vi "Build DB Connection String.vi"(8 "Error In":errorcluster) -> (0 "Error Out":errorcluster, 2 "Database Connection String":string)   [LabVIEW 2013, in "VIChallenge.lvlib"]
uses:
  VIChallenge.lvlib
  <vilib>/Utility/config.llb/Read Key (String).vi
  <vilib>/Utility/config.llb/NI_LVConfig.lvlib
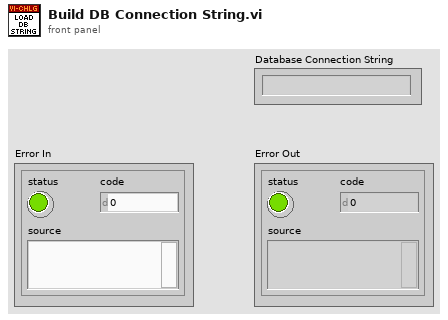
[diagram p1: front panel]
types:
  T1 = typedef "NI_LVConfig.lvlib/Config Data RefNum.ctl" = refnum<k1>
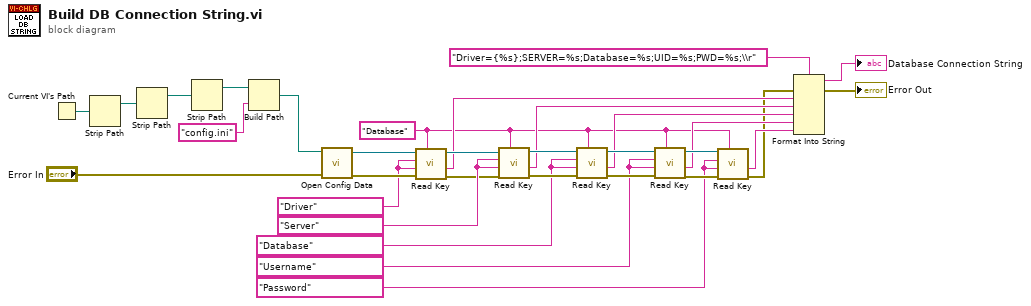
[diagram p0: block diagram]
diagram:
  w8 = "Password"
  w26 = "Username"
  w27 = "Database"
  w28 = "Server"
  w29 = "Driver"
  w3 = "Database" ("section")
  n1 = Current VI's Path() -> (path=w2:path)
  n2 = Strip Path(path=w2) -> (stripped path=w1:path)  [unwired: 1 out]
  n3 = Strip Path(path=w1) -> (stripped path=w20:path)  [unwired: 1 out]
  n4 = Strip Path(path=w20) -> (stripped path=w19:path)  [unwired: 1 out]
  n5 = Build Path(base path=w19, name or relative path="config.ini") -> (appended path=w17:path)
  n6 = call <vilib>:"Open Config Data.vi"("error in (no error)"="Error In", "configuration file path"=w17) -> ("error out"=w32:errorcluster, "refnum"=w22:T1)  [unwired: 7 in, 1 out]
  n7 = call-poly <vilib>:"Read Key.vi"("section"=w3, "error in (no error)"=w32, "default value"=w29, "key"=w29, "refnum"=w22) -> ("error out"=w23:errorcluster, "value"=w12:string, "refnum out"=w21:T1)  [unwired: 3 in, 1 out]
  n8 = call-poly <vilib>:"Read Key.vi"("section"=w3, "error in (no error)"=w23, "default value"=w28, "key"=w28, "refnum"=w21) -> ("error out"=w31:errorcluster, "value"=w11:string, "refnum out"=w25:T1)  [unwired: 3 in, 1 out]
  n9 = call-poly <vilib>:"Read Key.vi"("section"=w3, "error in (no error)"=w31, "default value"=w27, "key"=w27, "refnum"=w25) -> ("error out"=w30:errorcluster, "value"=w10:string, "refnum out"=w24:T1)  [unwired: 3 in, 1 out]
  n10 = call-poly <vilib>:"Read Key.vi"("section"=w3, "error in (no error)"=w30, "default value"=w26, "key"=w26, "refnum"=w24) -> ("error out"=w14:errorcluster, "value"=w9:string, "refnum out"=w15:T1)  [unwired: 3 in, 1 out]
  n11 = call-poly <vilib>:"Read Key.vi"("section"=w3, "error in (no error)"=w14, "default value"=w8, "key"=w8, "refnum"=w15) -> ("error out"=w6:errorcluster, "value"=w7:string)  [unwired: 3 in, 2 out]
  n12 = Format Into String(format string="Driver={%s};SERVER=%s;Database=%s;UID=%s;PWD=%s;\\r", error in=w6, w12, w11, w10, w9, w7) -> (resulting string=→"Database Connection String":string, error out=→"Error Out":errorcluster)  [unwired: 1 in]
